vi "subtract.vi"(8 "error in (no error)":errorcluster, 10 "subtrahend":refnum<class "SpaceVector.lvclass">, 11 "SpaceVector in":refnum<class "SpaceVector.lvclass">) -> (0 "error out":errorcluster, 3 "SpaceVector out":refnum<class "SpaceVector.lvclass">)   [LabVIEW 2010, in "SpaceVector.lvclass"]
uses:
  SpaceVector.lvclass
  SpaceVector.lvclass/SpaceVector.ctl
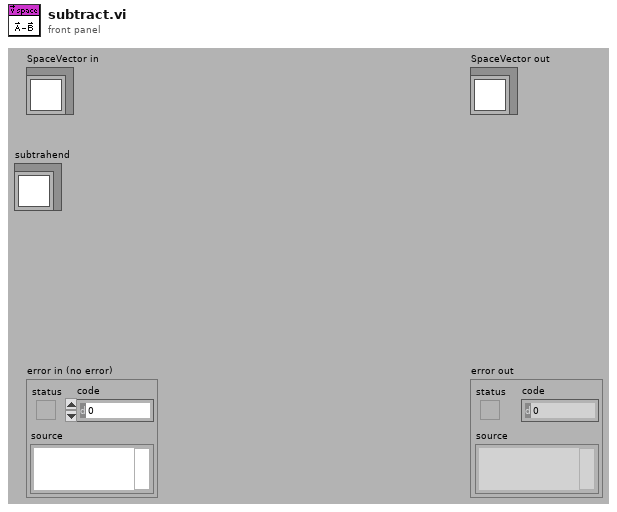
[diagram p1: front panel]
types:
  T1 = typedef "space_vector_array.ctl" = dbl[unit][]
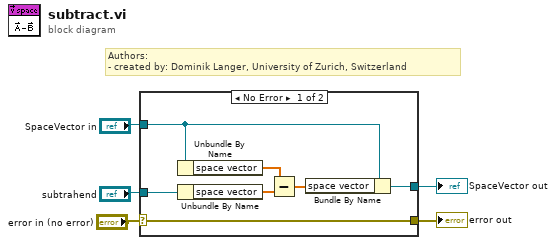
[diagram p0: block diagram]
diagram:
  # "Authors: \n- created by: Dominik Langer, University of Zurich, Switzerland"
  n1 = case shown="No Error" "error in (no error)" {
    selector: "error in (no error)" -> [w12 w14]
    tunnel: [w12 w14] -> w4
    tunnel: [w7 w13] -> w2
    tunnel: "SpaceVector in" -> [w8 w13]
    tunnel: "subtrahend" -> [w11 _]
    frame No Error {
      n2 = Unbundle By Name(w8) -> ("space vector"=w10:T1)
      n3 = Unbundle By Name(w11) -> ("space vector"=w9:T1)
      n4 = Subtract(x=w10, y=w9) -> (x-y=w6:T1)
      n5 = Bundle By Name(cluster=w8, "space vector"=w6) -> (w7:refnum<class "SpaceVector.lvclass">)
    }
    frame Error {
    }
  }
  "error out" <- w4
  "SpaceVector out" <- w2
